vi "test_fast_PID_chain3.vi"() -> ()   [LabVIEW 2013]
uses:
  Scope5782/Scope/controls/Memory block.ctl
  <vilib>/rvi/FXPMathLib/FxpConvert/subVIs/nifxpmath_Convert_SimConfig.ctl
  <vilib>/fxp/LVFixedPointQuantizationPolicyTypeDef.ctl
  <vilib>/fxp/LVFixedPointOverflowPolicyTypeDef.ctl
  <vilib>/rvi/FXPMathLib/FxpConvert/simVIs/DllFxpConvertTemp_sub.vi
  <vilib>/rvi/FXPMathLib/FxpConvert/XNode/nifxpmath_Convert.xnode
  <vilib>/measure/NI_MABase.lvlib
panel:
  out "Waveform Graph 4":i16[](graph)
  out "Waveform Graph 3":dbl[][](graph)
  out "Waveform Graph 2":dbl[](graph)
  out "Waveform Graph":dbl[](graph)
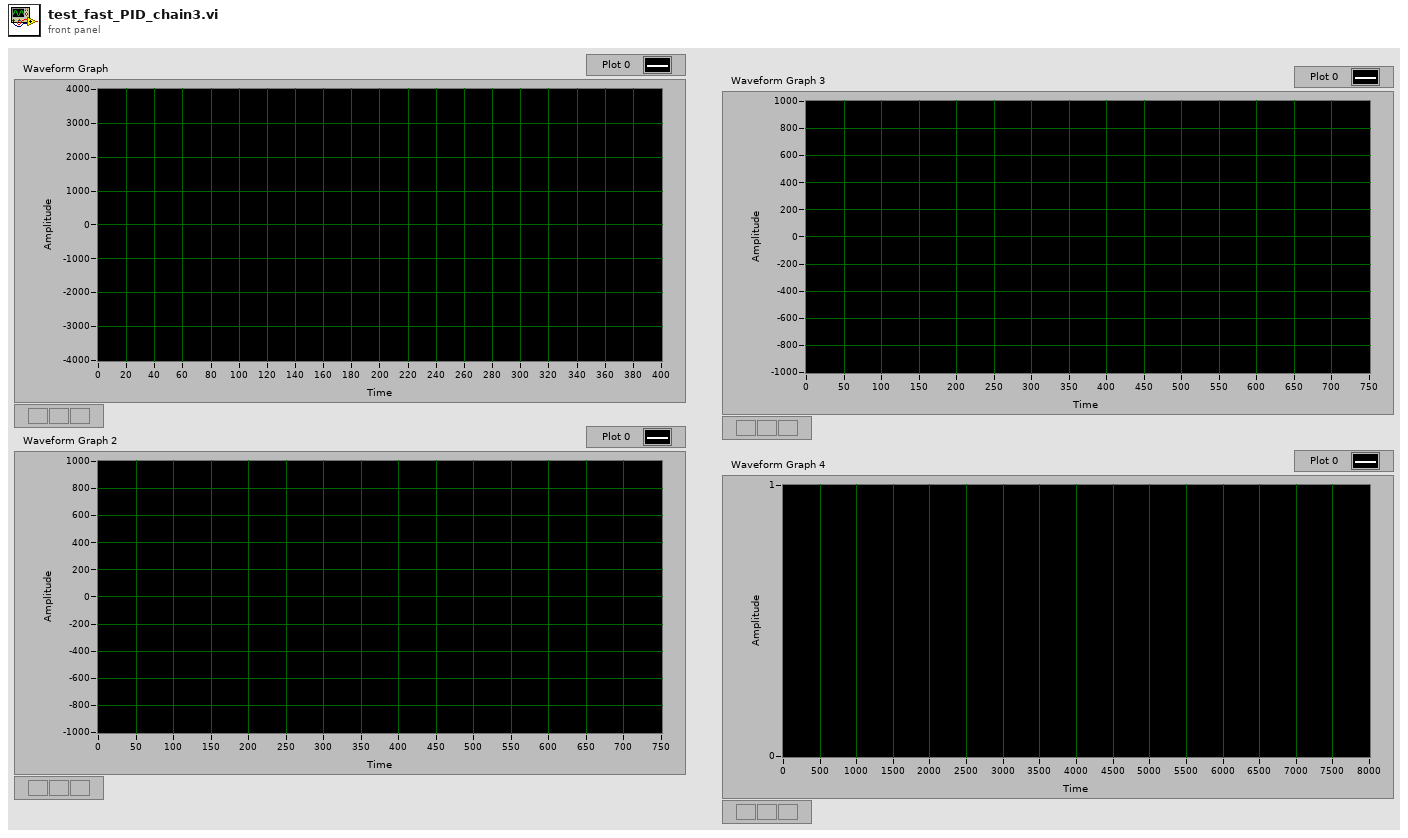
[diagram p1: front panel]
types:
  T1 = typedef "Memory block.ctl" = enum16{"Setpoint", "Beam"}
  T2 = cluster{"frequency":dbl, "amplitude":dbl, "phase":dbl}[]
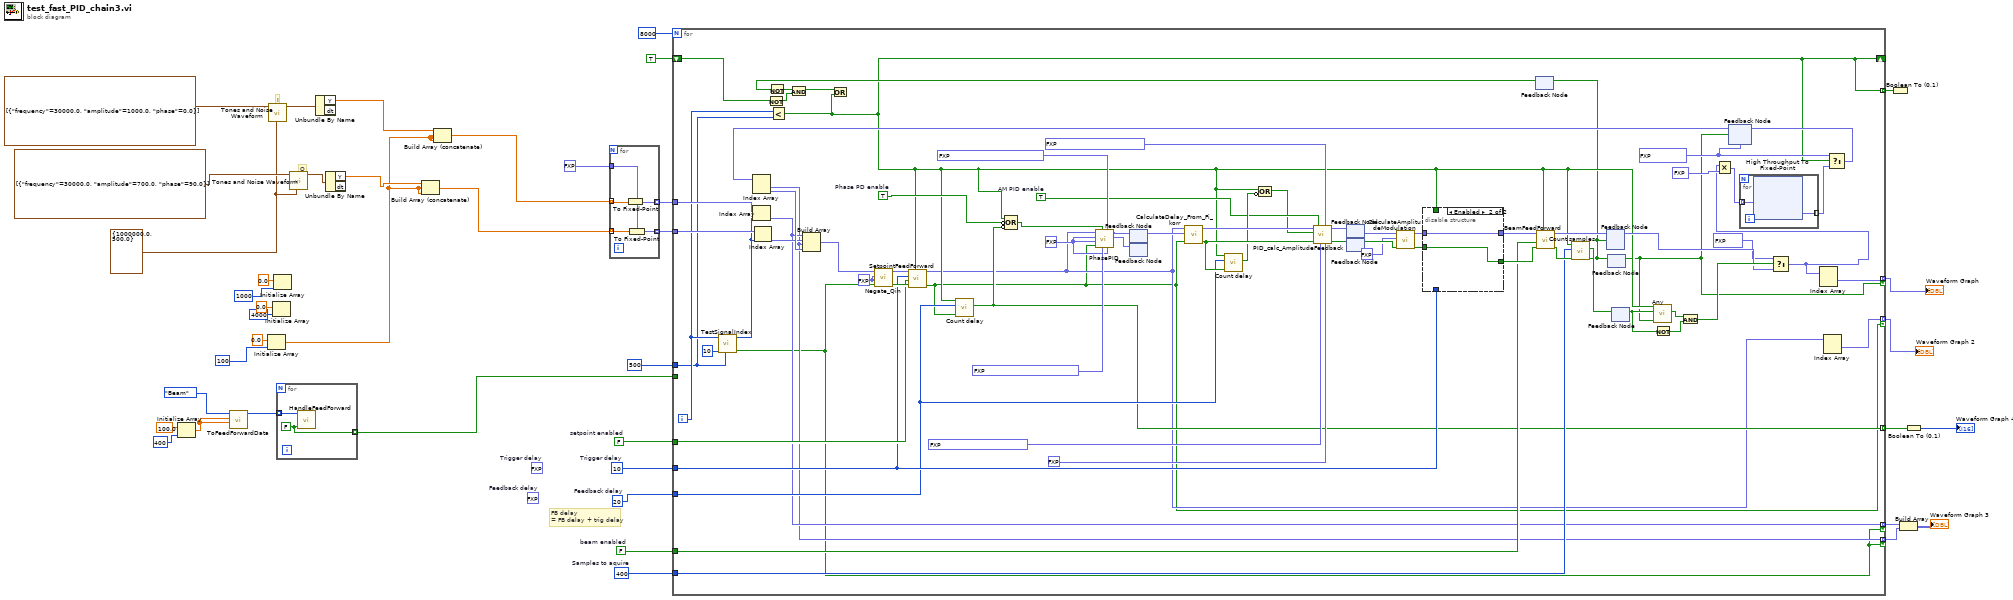
[diagram p0: block diagram]
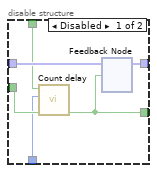
[diagram p2: hidden frame]
diagram:
  (unwired) fxp<+/-,16,16> 10.0  # Feedback delay
  (unwired) fxp<+/-,16,16> 25.0  # Trigger delay
  w34 = FALSE  # beam enabled
  w35 = u32 400  # Samples to aquire
  w36 = FALSE  # setpoint enabled
  w5 = u32 20  # Feedback delay
  w37 = u32 10  # Trigger delay
  w32 = cluster{"Fs":dbl, "#s":dbl} {"Fs"=1000000.0, "#s"=500.0} ("sampling info")
  # "Q"
  # "I"
  # "FB delay\n= FB delay + trig delay"
  n1 = Initialize Array(100.0 ("element"), 400 ("dimension size")) -> (w12:dbl[])
  n2 = call "ToFeedForwardData.vi"("values Q"=w12, "values I"=w12, "Memory block"=Memory_block."Beam") -> ("Data"=w16:u64[])  [unwired: 8 in]
  n3 = Initialize Array(0.0 ("element"), 100 ("dimension size")) -> (w6:dbl[])
  n4 = call <vilib>:"Tones and Noise Waveform.vi"("sampling info"=w32, "tones"=T2 [{"frequency"=30000.0, "amplitude"=1000.0, "phase"=0.0}]) -> ("signal out"=w39:waveform(dbl))  [unwired: 8 in, 1 out]
  n5 = Initialize Array(0.0 ("element"), 4000 ("dimension size")) -> ()  [unwired: 1 out]
  n6 = Initialize Array(0.0 ("element"), 1000 ("dimension size")) -> ()  [unwired: 1 out]
  n7 = for {
    tunnel: w16 -> [w43] mode=indexing
    tunnel: [w42] -> w9 mode=indexing
    w42 = FALSE ("timed out")
    n8 = call "HandleFeedForward.vi"("timed out"=w42, "Value"=w43) -> ()  [unwired: 10 in]
  }
  n9 = call <vilib>:"Tones and Noise Waveform.vi"("sampling info"=w32, "tones"=T2 [{"frequency"=30000.0, "amplitude"=700.0, "phase"=90.0}]) -> ("signal out"=w29:waveform(dbl))  [unwired: 8 in, 1 out]
  n10 = Unbundle By Name(w39) -> ("Y"=w25:dbl[])  [unwired: 1 out]
  n11 = Unbundle By Name(w29) -> ("Y"=w24:dbl[])  [unwired: 1 out]
  n12 = Build Array (concatenate)(w24, w6, w6) -> (w22:dbl[])
  n13 = Build Array (concatenate)(w25, w6, w6) -> (w17:dbl[])
  n14 = for {
    tunnel: w22 -> [w47] mode=indexing
    tunnel: fxp<+/-,16,14> 0.0 ("fixed-point type") -> [w48]
    tunnel: [w46] -> w38 mode=indexing
    tunnel: w17 -> [w44] mode=indexing
    tunnel: [w45] -> w21 mode=indexing
    n15 = To Fixed-Point(number=w44) -> (fixed-point=w45:fxp<+/-,16,14>)  [unwired: 1 in]
    n16 = To Fixed-Point(fixed-point type=w48, number=w47) -> (fixed-point=w46:fxp<+/-,16,14>)
  }
  n17 = for {
    N: 8000 -> [_]
    tunnel: w38 -> [w121]
    tunnel: w5 -> [w75]
    tunnel: w37 -> [w82]
    tunnel: w36 -> [w83]
    tunnel: w35 -> [w81]
    tunnel: w34 -> [w79]
    tunnel: w21 -> [w120]
    shift-right: [w59] -> _
    shift-left: TRUE -> [w114]
    tunnel: [w59] -> w18 mode=indexing
    tunnel: [w65] -> w11 mode=indexing if=w50
    tunnel: [w64] -> w10 mode=indexing if=w50
    tunnel: w9 -> [_]
    tunnel: 500 ("initial delay") -> [w71]
    tunnel: [w66] -> w4 mode=indexing if=w54
    tunnel: [w56] -> w3 mode=indexing
    tunnel: [w53] -> w1 mode=indexing if=w49
    i -> [w116]
    w63 = TRUE  # AM PID enable
    w62 = TRUE  # Phase PD enable
    w84 = fxp<+/-,16,14> 0.0 ("DC offset chan 1")
    w107 = fxp<+/-,16,14>[] [0.0, 0.0]
    w87 = fxp<+/-,32,4> 0.0 ("Fi_start")
    n18 = call "TestSignalIndex.vi"("initial delay"=w71, "cycles per sample"=10, "index"=w116) -> ("valid out"=w50:bool, "array index"=w109:i32)  [unwired: 7 in]
    n19 = Index Array(array=w120, index=w109) -> (element=w65:fxp<+/-,16,14>)
    n20 = Index Array(array=w121, index=w109) -> (element=w110:fxp<+/-,16,14>)
    n21 = Not(x=w114) -> (.not. x?=w112:bool)
    n22 = Less?(x=w116, y=w71) -> (x < y?=w59:bool)
    n23 = feedback #1() -> (w103:fxp<+/-,32,4>)  [unwired: 1 in]
    n24 = feedback #2() -> ()  [unwired: 2 in]
    n25 = feedback #3() -> (w77:fxp<+/-,16,14>[])  [unwired: 1 in]
    n26 = feedback #4() -> (w101:bool)  [unwired: 1 in]
    n27 = call "CalculateAmplitudeModulation.vi"("input valid"=w101, "AM_factor"=fxp<+/-,16,2> 1.0, "Data in"=w77) -> ("output valid"=w96:bool, "Data out"=w102:fxp<+/-,16,14>[])  [unwired: 7 in]
    n28 = disable-structure shown="Enabled" {
      disable-tunnel: w102 -> [w152 w154]
      disable-tunnel: [w151 w154] -> w100
      disable-tunnel: [w150 w153] -> w98
      disable-tunnel: w96 -> [w149 w153]
      disable-tunnel: w82 -> [w148 _]
      disable-tunnel: w59 -> [w147 _]
      frame Disabled {
        n29 = call "Count delay.vi"("input valid"=w149, "Count to skip"=w148, "Reset"=w147) -> ("output valid"=w150:bool)  [unwired: 7 in, 1 out]
        n30 = feedback #5() -> (w151:fxp<+/-,16,14>[])  [unwired: 1 in]
        n31 = feedback-in #5(w152, w150) -> ()
      }
      frame Enabled {
      }
    }
    n32 = feedback #6() -> (w115:bool)  [unwired: 1 in]
    n33 = Not(x=w115) -> (.not. x?=w113:bool)
    n34 = And(x=w113, y=w112) -> (x .and. y?=w111:bool)
    n35 = Or(x=w111, y=w59) -> ()  [unwired: 1 out]
    n36 = call "BeamFeedForward.vi"("Reset"=w59, "input valid"=w98, "beam enabled"=w79, "Data in"=w100) -> ("output valid"=w94:bool, "Data out"=w99:fxp<+/-,16,14>[])  [unwired: 6 in]
    n37 = call "Count samples.vi"("input valid"=w94, "number to count"=w81, "Reset"=w59) -> ("output valid"=w57:bool, "counting"=w60:bool)  [unwired: 7 in]
    n38 = feedback-in #6(w57) -> ()
    n39 = feedback #7() -> (w69:fxp<+/-,16,14>[])  [unwired: 1 in]
    n40 = feedback-in #7(w99, w57) -> ()
    n41 = feedback #8() -> (w54:bool)  [unwired: 1 in]
    n42 = feedback-in #8(w57) -> ()
    n43 = feedback #9() -> (w93:bool)  [unwired: 1 in]
    n44 = feedback-in #9(w60) -> ()
    n45 = call "Any.vi"("input valid"=w54, "Value"=w93, "Reset"=w59) -> ("Any?"=w92:bool)  [unwired: 7 in, 1 out]
    n46 = Not(x=w93) -> (.not. x?=w91:bool)
    n47 = And(x=w92, y=w91) -> (x .and. y?=w70:bool)
    n48 = feedback #10(w107) -> (w118:fxp<+/-,16,14>[])
    n49 = Index Array(array=w118) -> (element #1=w64:fxp<+/-,16,14>, element #2=w117:fxp<+/-,16,14>)  [unwired: 2 in]
    n50 = Build Array(w65, w110, w64, w117) -> (w52:fxp<+/-,16,14>[])
    n51 = call "Negate_Qin.vi"("valid in"=w50, "DC offset chan 1"=w84, "DC offset chan 0"=w84, "Data in"=w52) -> ("valid out"=w104:bool, "Data out"=w78:fxp<+/-,16,14>[])  [unwired: 6 in]
    n52 = call "SetpointFeedForward.vi"("Reset"=w59, "input valid"=w104, "setpoint enabled"=w83, "Samples to skip"=w82, "Data in"=w78) -> ("output valid"=w49:bool, "Data out"=w51:fxp<+/-,16,14>[])  [unwired: 5 in]
    n53 = call "Count delay.vi"("input valid"=w49, "Count to skip"=w75, "Reset"=w59) -> ("count done?"=w56:bool)  [unwired: 7 in, 1 out]
    n54 = Compound Arithmetic op=OR(w59, invert w62, invert w56) -> (w61:bool)
    n55 = call "PhasePID.vi"("Kd/Tau"=w87, "Ki*Tau"=fxp<+/-,32,4> 0.004999998956918716, "Kp"=fxp<+/-,32,4> 0.006000000983476639, "Reset"=w61, "input valid"=w49, "Fi_delta"=w87, "Fi_start"=w87, "Data in"=w51) -> ("Fi_korr"=w105:fxp<+/-,32,4>, "Fi_korr PID"=w106:fxp<+/-,32,4>)  [unwired: 1 in, 1 out]
    n56 = feedback-in #1(w106) -> ()
    n57 = feedback-in #2(w105) -> ()
    n58 = call "CalculateDelay_From_Fi_korr.vi"("input valid"=w49, "fi_korr"=w103, "Data in"=w51) -> ("output valid"=w76:bool, "Data out"=w95:fxp<+/-,16,14>[])  [unwired: 7 in]
    n59 = call "Count delay.vi"("input valid"=w76, "Count to skip"=w75, "Reset"=w59) -> ("count done?"=w74:bool)  [unwired: 7 in, 1 out]
    n60 = Compound Arithmetic op=OR(w59, invert w74) -> (w55:bool)
    n61 = call "PID_calc_AmplitudeFeedback.vi"("Kd/Tau"=fxp<+/-,32,6> 0.0 ("Data"), "Ki*Tau"=fxp<+/-,32,6> 0.0010000020265579224 ("Data"), "Kp"=fxp<+/-,32,6> 0.040000006556510925 ("Data"), "Enabled"=w63, "input valid"=w76, "Reset"=w55, "Data in"=w95) -> ("output valid"=w58:bool, "data out"=w97:fxp<+/-,16,14>[])  [unwired: 1 in, 2 out]
    n62 = feedback-in #3(w97) -> ()
    n63 = feedback-in #4(w58) -> ()
    n64 = Select(t=fxp<+/-,16,14>[] [0.0, 0.0], s=w70, f=w69) -> (s? t:f=w67:fxp<+/-,16,14>[])
    n65 = Multiply(x=w67, y=fxp<+/-,16,14> 0.25 ("Q out")) -> (x*y=w73:fxp<+/-,32,28>[])
    n66 = for {
      tunnel: w73 -> [w124] mode=indexing
      tunnel: [w123] -> w72 mode=indexing
      n67 = xnode "High Throughput To Fixed-Point"("x"=w124) -> ("y"=w123:fxp<+/-,16,14>)
    }
    n68 = Index Array(array=w67) -> (element #1=w66:fxp<+/-,16,14>)  [unwired: 2 in, 1 out]
    n69 = Index Array(array=w51) -> (element #1=w53:fxp<+/-,16,14>)  [unwired: 2 in, 1 out]
    n70 = Select(t=w107, s=w59, f=w72) -> (s? t:f=w108:fxp<+/-,16,14>[])
    n71 = feedback-in #10(w108, w54) -> ()
  }
  "Waveform Graph" <- w4
  "Waveform Graph 2" <- w1
  n72 = Boolean To (0,1)(Boolean=w18) -> ()  [unwired: 1 out]
  n73 = Build Array(w11, w10) -> (→"Waveform Graph 3":fxp<+/-,16,14>[][])
  n74 = Boolean To (0,1)(Boolean=w3) -> (0, 1=→"Waveform Graph 4":i16[])
